vi "BANDGAP DELTA POST TRIM - Write.vi"(8 "error in (no error)":errorcluster, 10 "BANDGAP DELTA POST TRIM":dbl[](array[numeric]), 11 "Globals in":refnum<class "TSM Context Data Access.lvclass">) -> (0 "error out":errorcluster, 3 "Globals out":refnum<class "TSM Context Data Access.lvclass">)   [LabVIEW 2019, in "TSM Context Data Access.lvclass"]
uses:
  TSM Context Data Access.lvclass
  TSM Context Data Access.lvclass/TSM Context Data Access.ctl
  <vilib>/NI_TestStand_SemiconductorModule/NI_TestStand_Semiconductor_Module.lvlibp
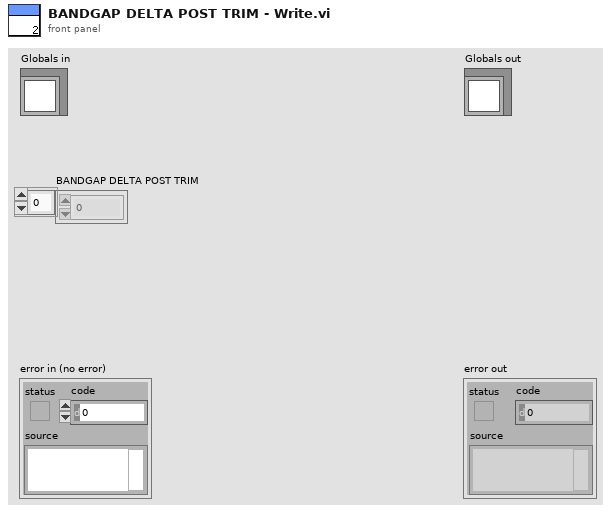
[diagram p1: front panel]
types:
  T1 = typedef "NI_TestStand_Semiconductor_Module.lvlibp/SemiconductorModuleContext.ctl" = refnum<k7>
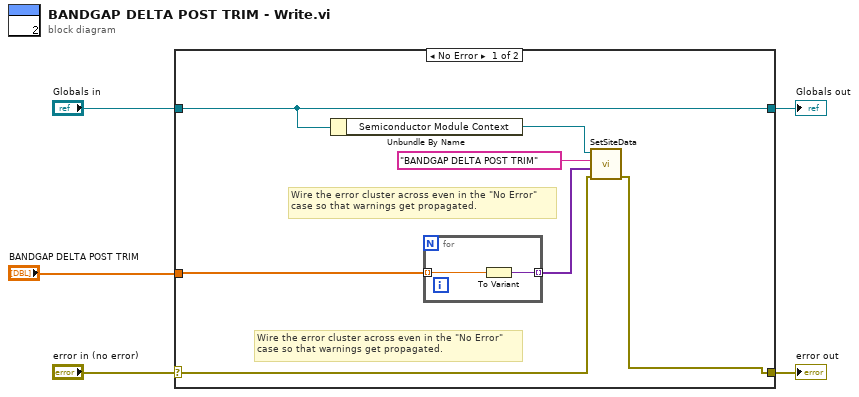
[diagram p0: block diagram]
diagram:
  n1 = case shown="No Error" "error in (no error)" {
    selector: "error in (no error)" -> [w10 w16]
    tunnel: [w9 w16] -> w4
    tunnel: [w8 w15] -> w2
    tunnel: "Globals in" -> [w8 w15]
    tunnel: "BANDGAP DELTA POST TRIM" -> [w7 _]
    frame No Error {
      # "Wire the error cluster across even in the \"No Error\"\ncase so that warnings get propagated."
      # "Wire the error cluster across even in the \"No Error\"\ncase so that warnings get propagated."
      n2 = Unbundle By Name(w8) -> ("Semiconductor Module Context"=w12:T1)
      n3 = for {
        tunnel: w7 -> [w14] mode=indexing
        tunnel: [w13] -> w6 mode=indexing
        n4 = To Variant(anything=w14) -> (Variant=w13:variant)
      }
      n5 = call <vilib>:"SetSiteData.vi"("error in (no error)"=w10, "Site Data"=w6, "Data Id"="BANDGAP DELTA POST TRIM", "Semiconductor Module Context"=w12) -> ("error out"=w9:errorcluster)  [unwired: 5 in, 1 out]
    }
    frame Error {
    }
  }
  "error out" <- w4
  "Globals out" <- w2
